vi "lv_mysql_conn_eof_packet.vi"(9 "Packet Metadata In":T1 {"Server Status" format="%.0x"}, 11 "TCPIP Data":u8[](array[numeric])) -> (1 "Packet Metadata Out":T1 {"Server Status" format="%.0x"})   [LabVIEW 2019]
uses:
  typedefs/ok_packet_metadata.ctl
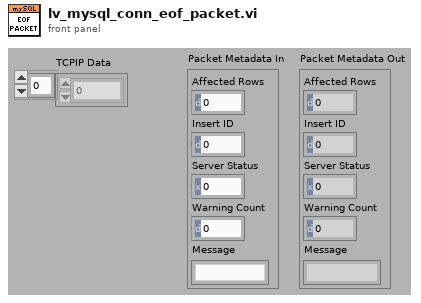
[diagram p1: front panel]
types:
  T1 = typedef "ok_packet_metadata.ctl" = cluster{"Affected Rows":u64, "Insert ID":u64, "Server Status":u16, "Warning Count":u16, "Message":string}
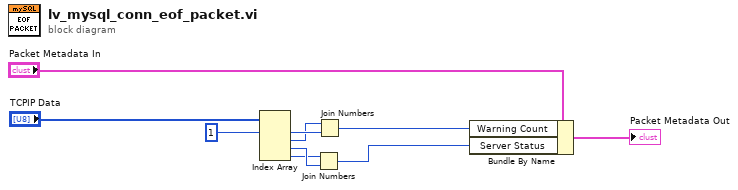
[diagram p0: block diagram]
diagram:
  n1 = Index Array(array="TCPIP Data", index #1=1 ("Start Index")) -> (element #1=w8:u8, element #2=w7:u8, element #3=w5:u8, element #4=w4:u8)  [unwired: 3 in]
  n2 = Join Numbers(hi=w4, lo=w5) -> ((hi.lo)=w3:u16)
  n3 = Join Numbers(hi=w7, lo=w8) -> ((hi.lo)=w6:u16)
  n4 = Bundle By Name(cluster="Packet Metadata In", "Warning Count"=w6, "Server Status"=w3) -> (→"Packet Metadata Out":T1)
